vi "Open.vi"(8 "error in (no error)":errorcluster, 11 "MelsecTCP in":refnum<class "DeltaTcp.lvclass">) -> (0 "error out":errorcluster, 3 "MelsecTCP out":refnum<class "DeltaTcp.lvclass">)   [LabVIEW 2020, in "HslCommunication.lvlib" / "DeltaTcp.lvclass"]
uses:
  DeltaTcp.lvclass
  D:/Project/Labview-Projects/General utility tool/Libraries/HslCommunication/Abstract PLC Controler/Abstract PLC Controler.lvclass
  EventLogger.lvlibp/1abvi3w/vi.lib/gpm_packages/@cs/event-logger/Source/Composed Log/Types/Log Level.ctl
  Abstract PLC Controler/Abstract PLC Controler.lvclass/Abstract PLC Controler.ctl
  DeltaTcp.lvclass/DeltaTcp.ctl
  D:/Project/Labview-Projects/General utility tool/Libraries/HslCommunication/_Dependenciecs/HslCommunication.dll
  _Dependenciecs/HslCommunication.dll
  Read series.vi
  Read ipAddress.vi
  Read port.vi
  Abstract PLC Controler/Abstract PLC Controler.lvclass
  EventLogger.lvlibp/Logger.lvclass
  EventLogger.lvlibp/1abvi3w/vi.lib/gpm_packages/@cs/event-logger/Source/Composed Log/Composed Log.lvlib
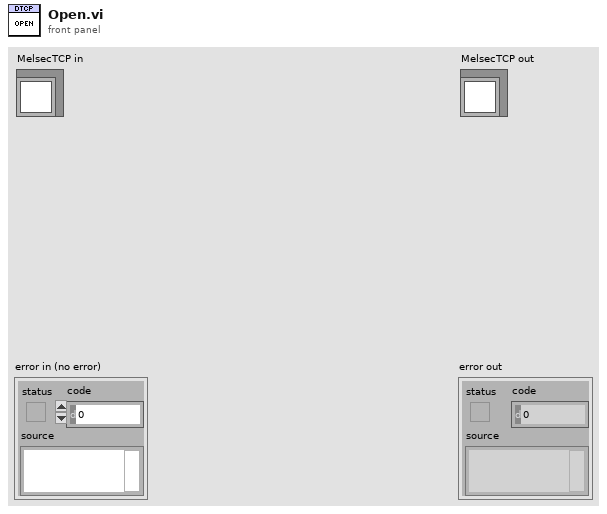
[diagram p1: front panel]
types:
  T1 = typedef "EventLogger.lvlibp/Composed Log.lvlib/Log Level.ctl" = enum16{"Debug", "Info", "Warning", "Error", "Critical"}
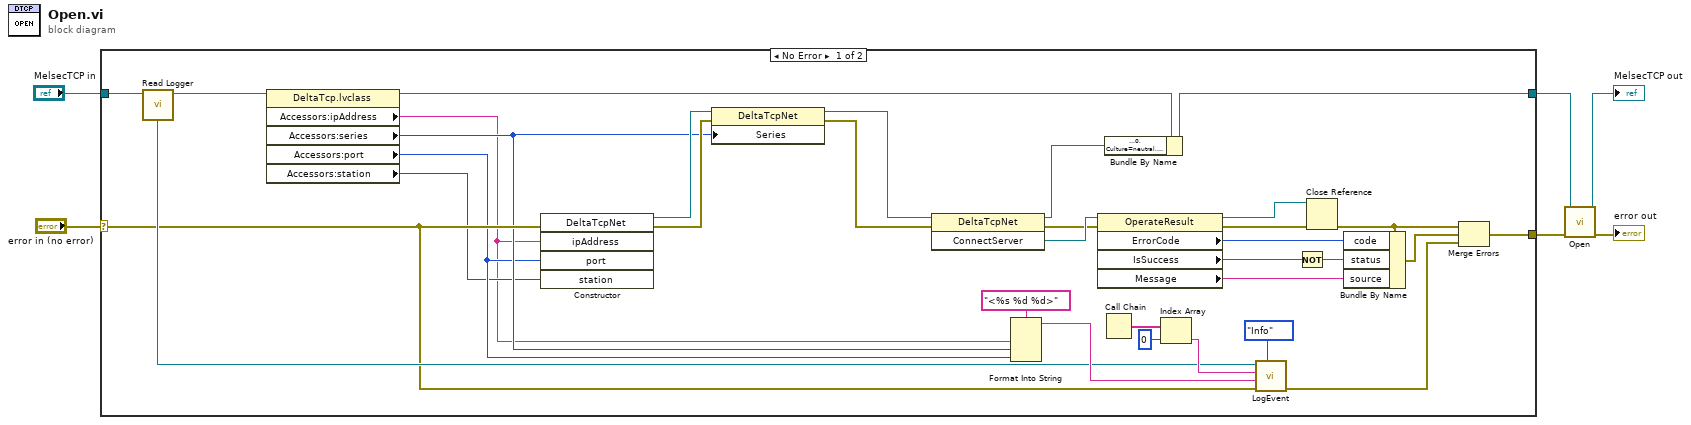
[diagram p0: block diagram]
diagram:
  n1 = case shown="No Error" "error in (no error)" {
    selector: "error in (no error)" -> [w18 w41]
    tunnel: "MelsecTCP in" -> [w39 w40]
    tunnel: [w38 w40] -> w2
    tunnel: [w32 w41] -> w4
    frame No Error {
      n2 = call "Read Logger.vi"("Abstract PLC Controler in"=w39) -> ("EventLogger.lvlibp:Logger.lvclass"=w19:refnum<class "Logger.lvclass">, "Abstract PLC Controler out"=w25:refnum<class "DeltaTcp.lvclass">)  [unwired: 9 in]
      n3 = property class="DeltaTcp.lvclass"(reference=w25) -> (reference out=w26:refnum<class "DeltaTcp.lvclass">, "Accessors:ipAddress"=w7:string, "Accessors:series"=w10:i32, "Accessors:port"=w9:i32, "Accessors:station"=w8:u8)  [unwired: 1 in, 1 out]
      n4 = constructor class="DeltaTcpNet"(error in=w18, "ipAddress"=w7, "port"=w9, "station"=w8) -> (reference out=w13:refnum<k24>, error out=w14:errorcluster)  [unwired: 2 in, 4 out]
      n5 = property class="DeltaTcpNet"(reference=w13, error in=w14, "Series"=w10) -> (reference out=w12:refnum<k24>, error out=w11:errorcluster)
      n6 = invoke class="DeltaTcpNet" method="ConnectServer"(reference=w12, error in=w11) -> (reference out=w15:refnum<k24>, error out=w29:errorcluster, "ConnectServer"=w31:refnum<k24>)  [unwired: 1 in]
      n7 = Format Into String(format string="<%s %d %d>", w7, w10, w9) -> (resulting string=w21:string)  [unwired: 2 in, 1 out]
      n8 = property class="OperateResult"(reference=w31, error in=w29) -> (reference out=w30:refnum<k24>, error out=w28:errorcluster, "ErrorCode"=w35:i32, "IsSuccess"=w27:bool, "Message"=w33:string)
      n9 = Call Chain() -> (call chain=w24:string[])
      n10 = Bundle By Name(cluster=w26, "reference"=w15) -> (w38:refnum<class "DeltaTcp.lvclass">)
      n11 = Index Array(array=w24, index=0) -> (element=w20:string)
      n12 = call "LogEvent.vi"("Event Level"=Log_Level."Info", "error in (no error)"=w18, "Data To Log"=w21, "SourceID"=w20, "Logger in"=w19) -> ("error out"=w17:errorcluster)  [unwired: 5 in, 1 out]
      n13 = Not(x=w27) -> (.not. x?=w34:bool)
      n14 = Close Reference(reference=w30, error in (no error)=w28) -> (error out=w36:errorcluster)
      n15 = Bundle By Name(cluster=w36, "code"=w35, "status"=w34, "source"=w33) -> (w37:errorcluster)
      n16 = Merge Errors(w36, w37, w17) -> (w32:errorcluster)
    }
    frame Error {
    }
  }
  n17 = call-parent "Open.vi"("error in (no error)"=w4, "MelsecTCP in"=w2) -> ("error out"=→"error out":errorcluster, "MelsecTCP out"=→"MelsecTCP out":refnum<class "DeltaTcp.lvclass">)  [unwired: 8 in]
